vi "03x check package version.vi"() -> ()   [LabVIEW 2018, in "LV-0mq-Julia_roundtrip-lib.lvlib"]
uses:
  LV-0mq-Julia_roundtrip-lib.lvlib
  Server or client state.ctl
  VersionNumber.ctl
  Commands.ctl
  jl-scripts path.vi
panel:
  out "LV client v":T1
  out "Jl server v":T1
  in  "next":bool
  out "current error":errorcluster
  out "final error":errorcluster
  out "short err code":u8
  in  "stop":bool
  out "ZMQ timeout":bool
  out "Julia script file path":path
  out "temporary script path":path
  out "Jl Server state":T2
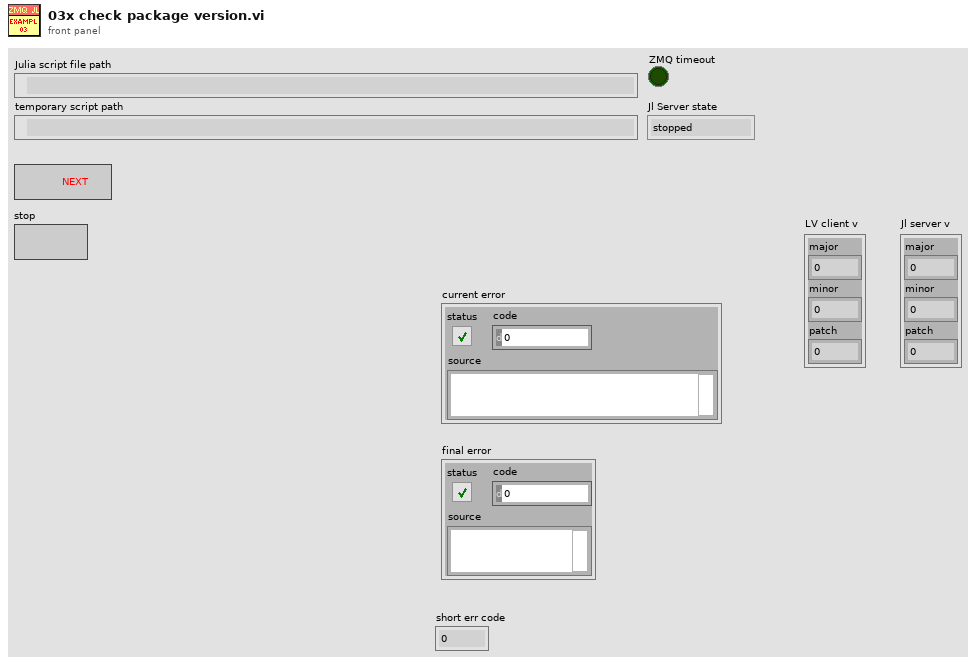
[diagram p1: front panel]
types:
  T1 = typedef "LV-0mq-Julia_roundtrip-lib.lvlib/VersionNumber.ctl" = cluster{"major":u16, "minor":u16, "patch":u16}
  T2 = typedef "LV-0mq-Julia_roundtrip-lib.lvlib/Server or client state.ctl" = enum16{"stopped", "running", "unknown"}
  T3 = typedef "LV-0mq-Julia_roundtrip-lib.lvlib/Commands.ctl" = enum16{"Start Jl-server & Init LV-client", "Send request & Get response ", "Stop Jl-server & Cleanup LV-client", "Cleanup LV-client", "Start Jl-server", "Stop Jl-server", "Init LV-Client", "Cleanup LV-Client", "(not allowed)", "Set LV Client state", "Set Jl Server state", "set ZMQ timeout", "read ZMQ timeout", "read-out state"}
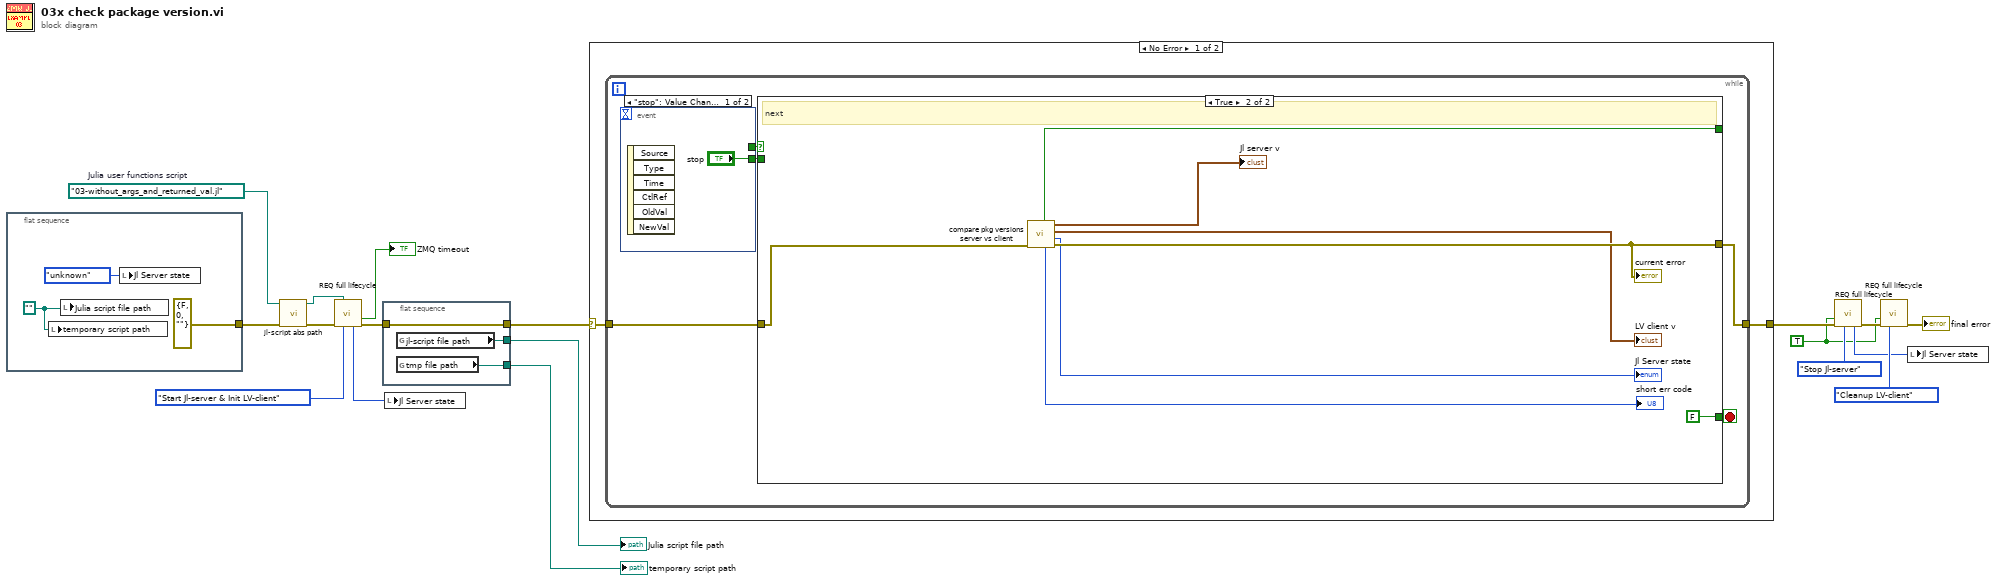
[diagram p0: block diagram]
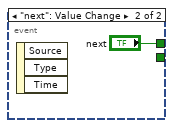
[diagram p2: hidden frame]
diagram:
  w4 = path "03-without_args_and_returned_val.jl"  # Julia user functions script
  w1 = TRUE ("Force command")
  n1 = flat-sequence {
    tunnel: [errorcluster {"status"=FALSE, "code"=0, "source"=""} ("error in (no error)")] -> w2
    frame #0 {
      w19 = path ""
      n2 = local write "temporary script path"(w19) -> ()
      n3 = local write "Julia script file path"(w19) -> ()
      n4 = local write "Jl Server state"(Server_or_client_state."unknown" ("Jl Server state out")) -> ()
    }
  }
  n5 = call "jl-script abs path.vi"("error in (no error)"=w2, "Julia user functions script"=w4) -> ("error out"=w5:errorcluster, "script abs path"=w6:path)  [unwired: 8 in]
  n6 = call "REQ full lifecycle.vi"("Julia user functions script"=w6, "error in"=w5, "command"=Commands."Start Jl-server & Init LV-client") -> ("timeout?"=→"ZMQ timeout":bool, "Jl Server state out"=w8:T2, "error out"=w7:errorcluster)  [unwired: 6 in, 4 out]
  n7 = flat-sequence {
    tunnel: [w24] -> w13
    tunnel: w7 -> [w24]
    tunnel: [w23] -> w11
    tunnel: [w22] -> w12
    frame #0 {
      n8 = global read "jl-scripts path.vi" "jl-script file path"() -> (w23:path)
      n9 = global read "jl-scripts path.vi" "tmp file path"() -> (w22:path)
    }
  }
  n10 = local write "Jl Server state"(w8) -> ()
  n11 = case shown="No Error" w13 {
    selector: w13 -> [w25 w44]
    tunnel: [w26 w44] -> w18
    frame No Error {
      n12 = while {
        tunnel: w25 -> [w30]
        tunnel: [w31] -> w26
        stop <- w28 stop-if-true
        n13 = event shown="[0] \"stop\": Value Change" {
          selector: _ -> [_ _]
          dyn-events: _ -> [_ _]
          timeout: _ -> [_ _]
          tunnel: [_ "next"] -> w29
          tunnel: ["stop" _] -> w27
          event "stop": Value Change {
            n14 = event-data() -> ()  [unwired: 1 in, 6 out]
          }
          event "next": Value Change {
            n15 = event-data() -> ()  [unwired: 1 in, 3 out]
          }
        }
        n16 = case shown="True" w29 {
          tunnel: [w35 w41] -> w31
          tunnel: w30 -> [w35 w42]
          tunnel: [w34 FALSE ("stop this VI only")] -> w28
          tunnel: w27 -> [w34 _]
          tunnel: [_ w38] -> _
          frame False {
            # "stop"
          }
          frame True {
            # "next"
            n17 = call "compare pkg versions server vs client.vi"("error in (no error)"=w42) -> ("error out"=w41:errorcluster, "Jl Server state out"=→"Jl Server state":T2, "Pkg v LV client"=→"LV client v":T1, "Pkg v Jl server"=→"Jl server v":T1, "return code"=→"short err code":u8, "timeout?"=w38:bool)  [unwired: 4 in, 1 out]
            "current error" <- w41
          }
        }
      }
    }
    frame Error {
    }
  }
  n18 = call "REQ full lifecycle.vi"("Force command"=w1, "error in"=w18, "command"=Commands."Stop Jl-server") -> ("Jl Server state out"=w10:T2, "error out"=w16:errorcluster)  [unwired: 6 in, 5 out]
  n19 = call "REQ full lifecycle.vi"("Force command"=w1, "error in"=w16, "command"=Commands."Cleanup LV-client") -> ("error out"=→"final error":errorcluster)  [unwired: 6 in, 6 out]
  n20 = local write "Jl Server state"(w10) -> ()
  "temporary script path" <- w12
  "Julia script file path" <- w11
